vi "Build Error Cluster.vi"(1 "String to Prepend to source (\"\")":string, 2 "code":i32) -> (0 "error out":errorcluster)   [LabVIEW 2012, in "TD Tools.lvlib"]
uses:
  TD Tools.lvlib
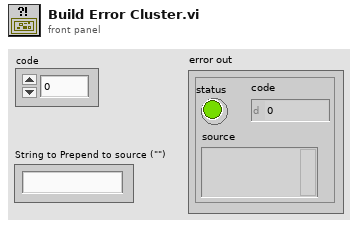
[diagram p1: front panel]
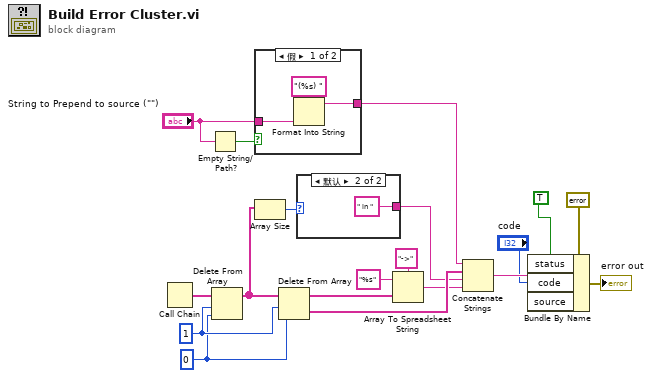
[diagram p0: block diagram]
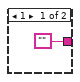
[diagram p2: hidden frame]
diagram:
  w15 = 0 ("索引")
  w16 = 1 ("长度")
  n1 = Call Chain() -> (call chain=w17:string[])
  n2 = Empty String/Path?(string/path="String to Prepend to source (\"\")") -> (empty?=w19:bool)
  n3 = Delete From Array(array=w17, length=w16, index=w15) -> (array with subset deleted=w8:string[])  [unwired: 1 out]
  n4 = case shown="假" w19 {
    tunnel: "String to Prepend to source (\"\")" -> [w21 w23]
    tunnel: [w20 w23] -> w11
    frame False {
      n5 = Format Into String(format string="(%s) " ("Format String"), w21) -> (resulting string=w20:string)  [unwired: 2 in, 1 out]
    }
    frame True {
    }
  }
  n6 = Array Size(array=w8) -> (size(s)=w7:i32)
  n7 = Delete From Array(array=w8, length=w16, index=w15) -> (deleted portion=w10:string[], array with subset deleted=w12:string[])
  n8 = case shown="默认" w7 {
    tunnel: ["" " in " ("Format String")] -> w6
    frame 1 {
    }
    frame Default {
    }
  }
  n9 = Array To Spreadsheet String(delimiter (Tab)="->", array=w12, 3:"%s" ("format string")) -> (spreadsheet string=w9:string)
  n10 = Concatenate Strings(w11, w10, w6, w9) -> (w5:string)
  n11 = Bundle By Name(cluster=errorcluster {"status"=FALSE, "code"=0, "source"=""} ("error out"), "status"=TRUE, "code"="code", "source"=w5) -> (→"error out":errorcluster)
